vi "Autonomous Independent.vi"() -> ()   [LabVIEW 2014]
doc: "This VI is called when autonomous begins, and will automatically be terminated when autonomous ends. You can carry out timed or sensor driven robot movement independently without needing to return to the caller."
uses:
  <vilib>/Rock Robotics/WPI/SafetyOutput/WPI_SafetyOutputConfigMenu.ctl
  <vilib>/Rock Robotics/WPI/Joystick/WPI_JoystickGetSetRefNum.vi
  <vilib>/Rock Robotics/Network Tables/SD Read Number.vi
  <vilib>/Rock Robotics/WPI/RobotDrive/WPI_RobotDriveGetSetRefNum.vi
  <vilib>/Rock Robotics/WPI/RobotDrive/WPI_RobotDriveArcadeDrive_Standard(NoSaturation).vi
panel:
  out "Current Movement, for debugging":T1 {"Y Joystick Value" scale=1.0..-1.0; "X Joystick Value" scale=-1.0..1.0}
  in  "Array of robot movements":T2(array[cluster]) {"Y Joystick Value" scale=1.0..-1.0; "X Joystick Value" scale=-1.0..1.0}
  # "Be sure to right-click and choose Data Operations>>Make Current Value default if you want to save the array values with the VI"
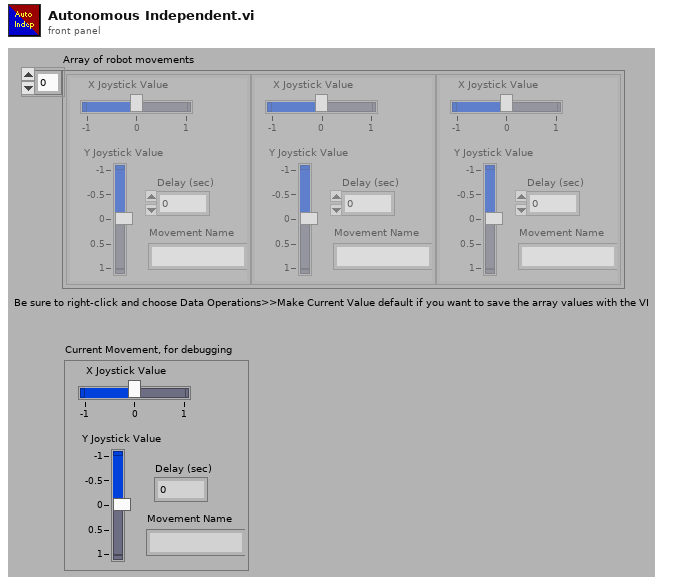
[diagram p1: front panel]
types:
  T1 = cluster{"X Joystick Value":dbl, "Y Joystick Value":dbl, "Delay (sec)":dbl, "Movement Name":string}
  T2 = cluster{"X Joystick Value":dbl, "Y Joystick Value":dbl, "Delay (sec)":dbl, "Movement Name":string}[]
  T3 = typedef "WPI_SafetyOutputConfigMenu.ctl" = enum16{"Enable", "Disable"}
  T4 = typedef "WPI_RobotDriveDevRef.ctl" = cluster{"DevStatus":errorcluster, "Motors[]":T5[], "Square Inputs":bool, "Max Output":dbl}
  T5 = typedef "WPI_MotorControlDeviceRef.ctl" = cluster{"DeviceStatus":errorcluster, "Type":T6, "PWM":cluster{"Controller":T7, "PWM Channel":T8, "DeadBand":T9}, "CAN":cluster{"Device Number":u8, "Control Mode":T10, "Semaphore":T11, "Max Vout":dbl, "TalonSRX Control Mode":T12}, "Invert":bool, "TransformRef":T13, "InvTransformRef":T13}
  T6 = typedef "WPI_MotorControlType.ctl" = enum16{"PWM", "CAN", "CANTalonSRX"}
  T7 = typedef "FPGA_TypedefDigitalModule.ctl" = enum16{"Controller 1"}
  T8 = typedef "FPGA_DIOPWMChannel.ctl" = enum8{"PWM 0", "PWM 1", "PWM 2", "PWM 3", "PWM 4", "PWM 5", "PWM 6", "PWM 7", "PWM 8", "PWM 9", "PWM MXP 0", "PWM MXP 1", "PWM MXP 2", "PWM MXP 3", "PWM MXP 4", "PWM MXP 5", "PWM MXP 6", "PWM MXP 7", "PWM MXP 8", "PWM MXP 9", "Invalid"}
  T9 = typedef "WPI_PWMDeadband.ctl" = cluster{"Name":string, "maxPositivePwm":i32, "minPositivePwm":i32, "centerPwm":i32, "maxNegativePwm":i32, "minNegativePwm":i32, "angularRange":u16}
  T10 = typedef "WPI_CANJaguar_ControlMode.ctl" = enum8{"Percent VBus", "Current", "Speed", "Position", "Voltage"}
  T11 = typedef "Semaphore RefNum" = refnum<k1>
  T12 = typedef "WPI_CANTalonSRX_APIControlMode.ctl" = enum8{"Percent VBus", "Speed", "Position", "Slave", "Unchanged / Invalid"}
  T13 = typedef "WPI_PWMTransform_ConPane.ctl" = refnum<vi>
  T14 = typedef "WPI_JoystickDevRef.ctl" = cluster{"Device":T15}
  T15 = typedef "WPI_JoystickDeviceEnum.ctl" = enum16{"USB 0", "USB 1", "USB 2", "USB 3", "USB 4", "USB 5"}
  T16 = typedef "WPI_GyroDevRef.ctl" = cluster{"DevStatus":errorcluster, "Analog Module":T17, "Analog Channel":T18, "Offset":dbl, "Gain (VoltsPerDegree/Second)":dbl}
  T17 = typedef "FPGA_TypedefAnalogModule.ctl" = enum16{"Controller 1"}
  T18 = typedef "FPGA_AIChannel.ctl" = enum8{"AI 0", "AI 1", "AI 2", "AI 3", "AI MXP 0", "AI MXP 1", "AI MXP 2", "AI MXP 3", "Invalid"}
  T19 = typedef "WPI_DigitalInputDevRef.ctl" = cluster{"DevStatus":errorcluster, "DIO Channel":T20, "Controller":T7}
  T20 = typedef "FPGA_DIOChannel.ctl" = enum8{"DIO 0", "DIO 1", "DIO 2", "DIO 3", "DIO 4", "DIO 5", "DIO 6", "DIO 7", "DIO 8", "DIO 9", "DIO MXP 0", "DIO MXP 1", "DIO MXP 2", "DIO MXP 3", "DIO MXP 4", "DIO MXP 5", "DIO MXP 6", "DIO MXP 7", "DIO MXP 8", "DIO MXP 9", "DIO MXP 10", "DIO MXP 11", "DIO MXP 12", "DIO MXP 13", "DIO MXP 14", "DIO MXP 15", "Invalid"}
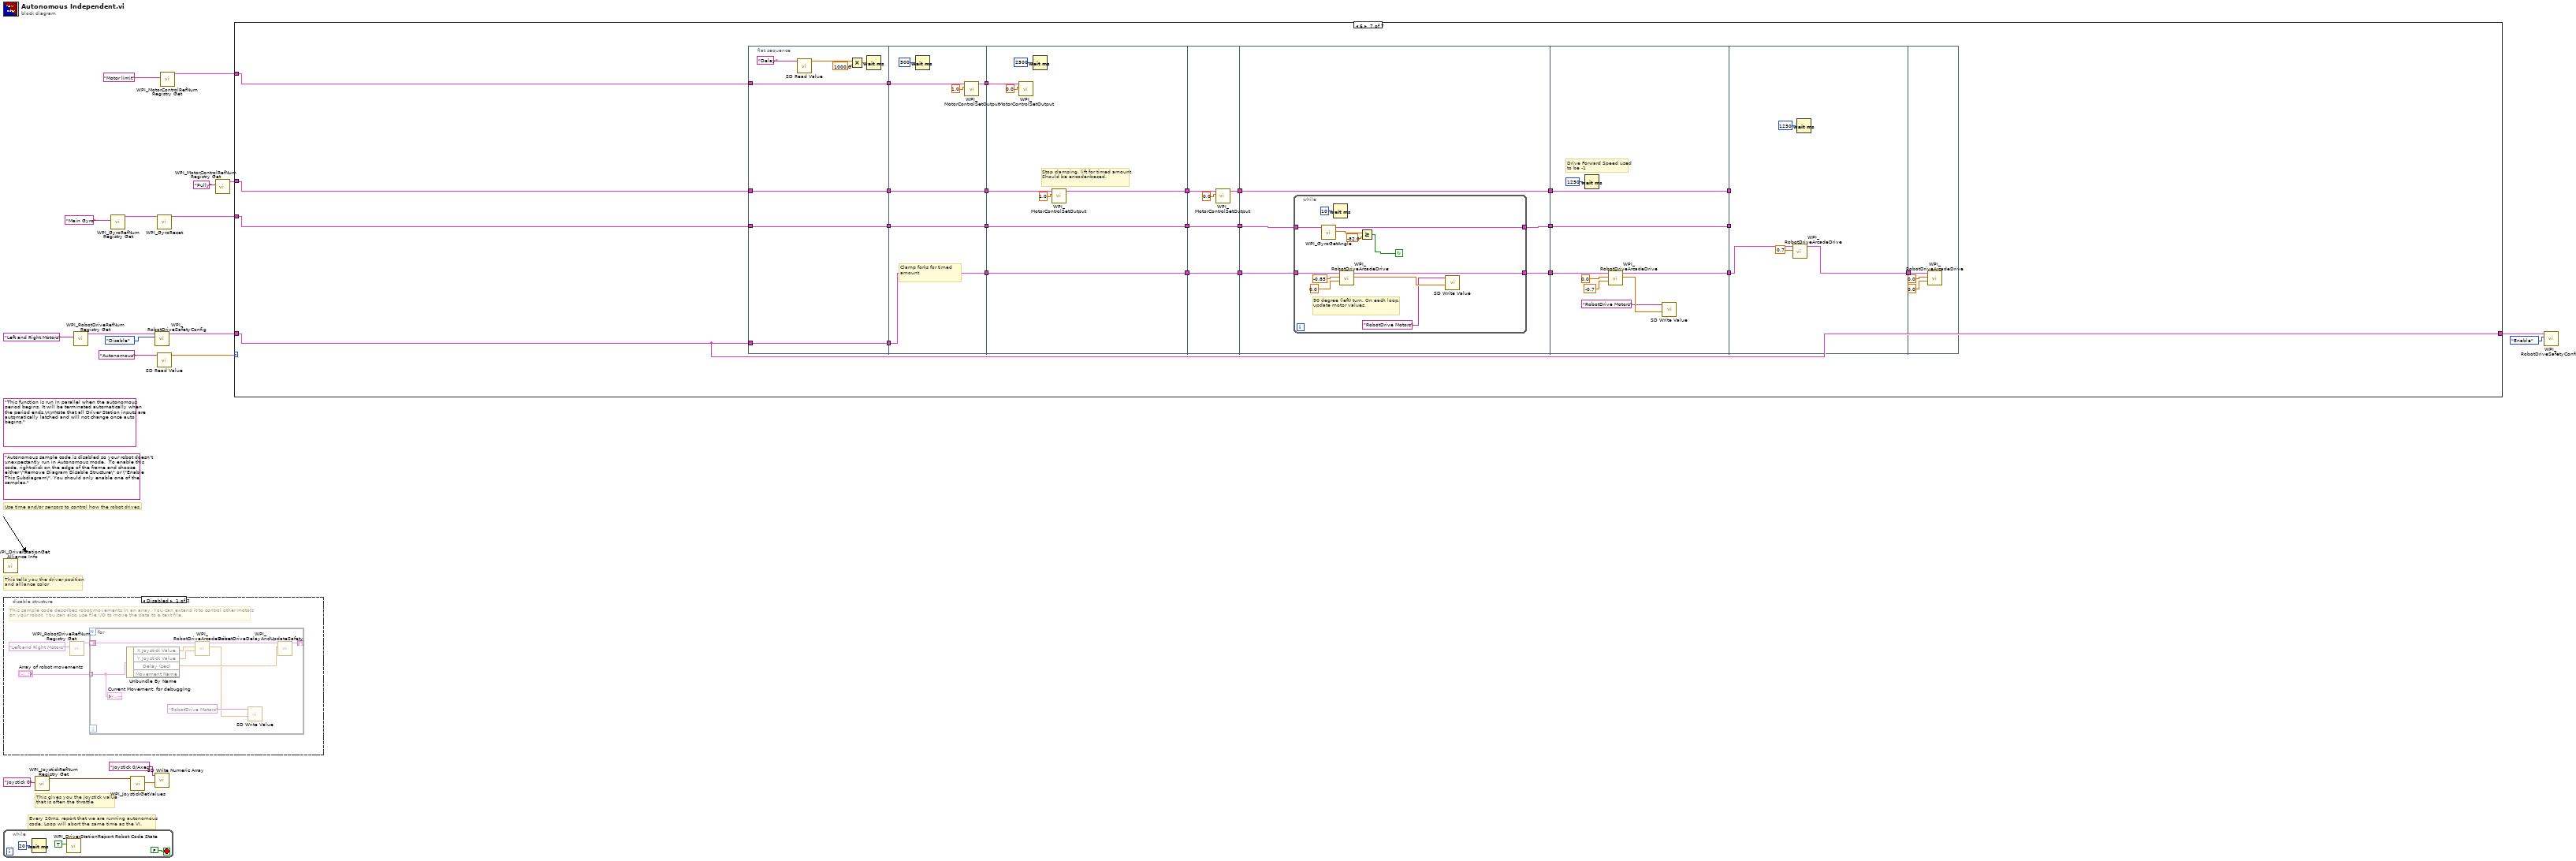
[diagram p0: block diagram]
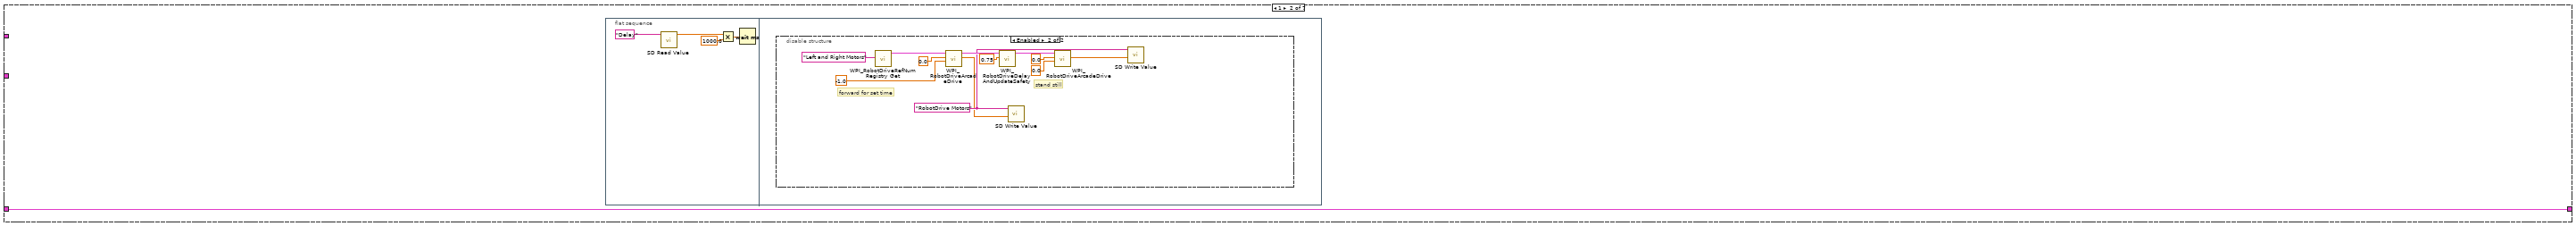
[diagram p3: hidden frame]
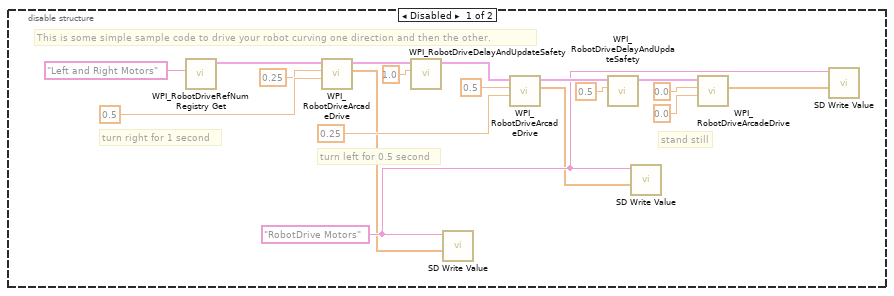
[diagram p4: hidden frame]
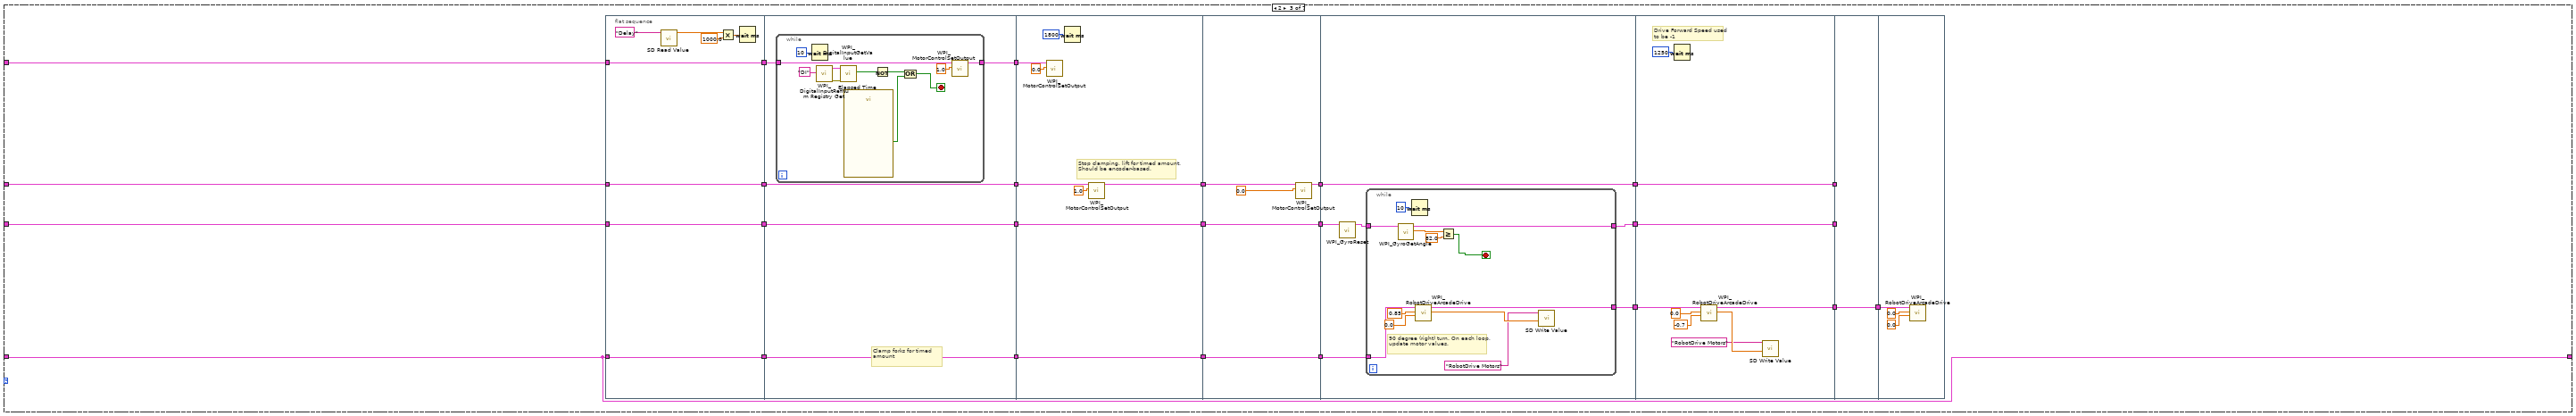
[diagram p5: hidden frame]
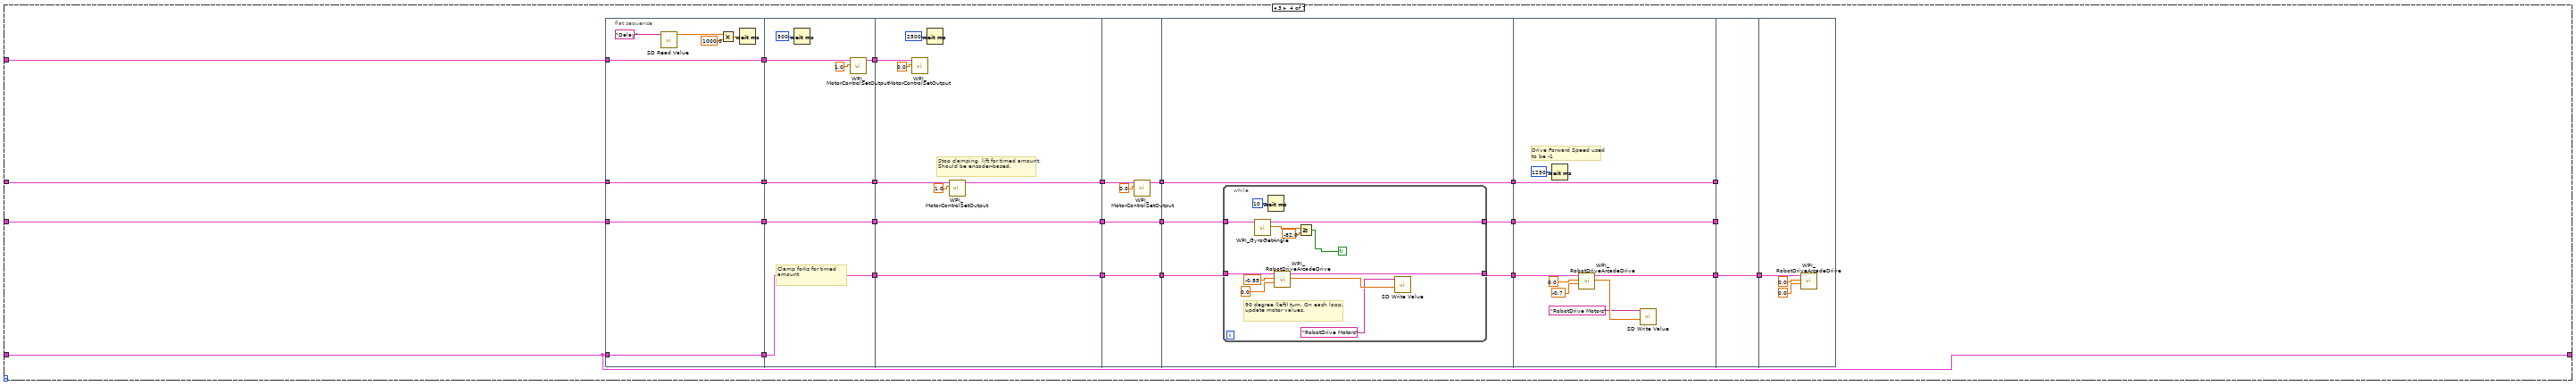
[diagram p6: hidden frame]
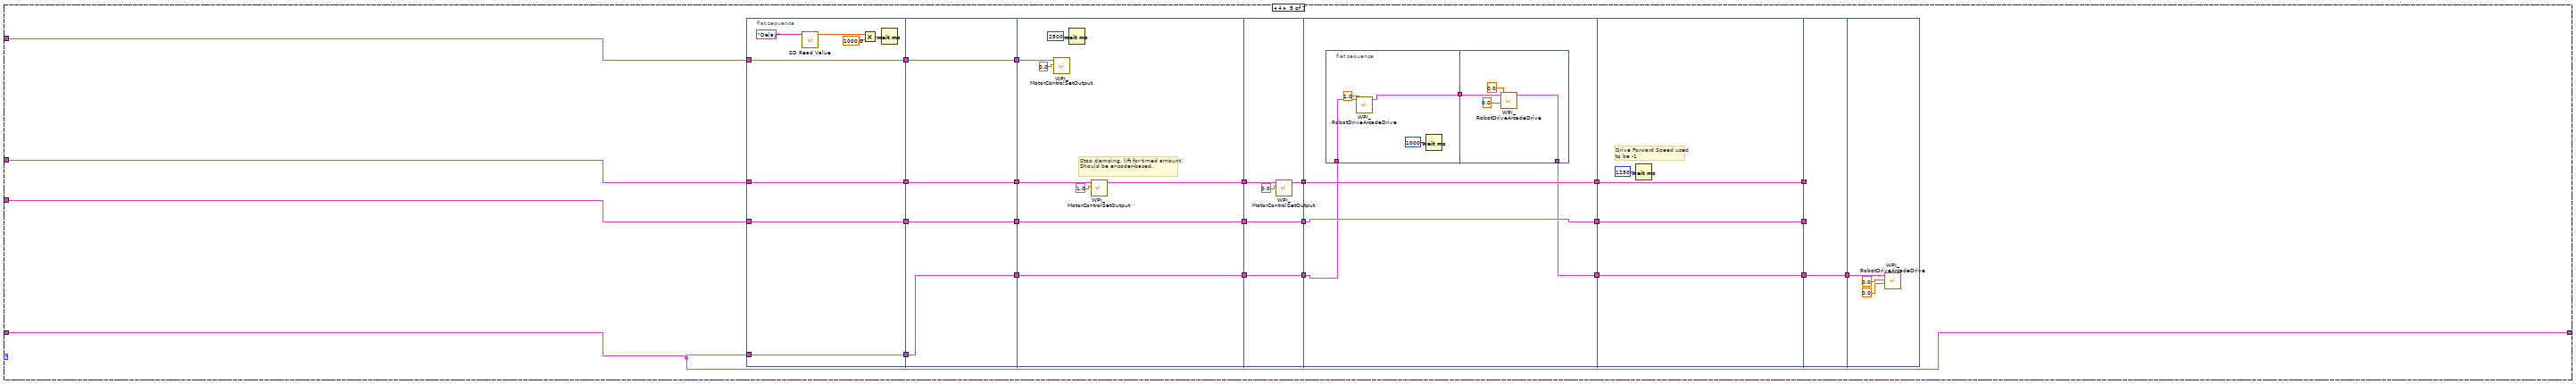
[diagram p7: hidden frame]
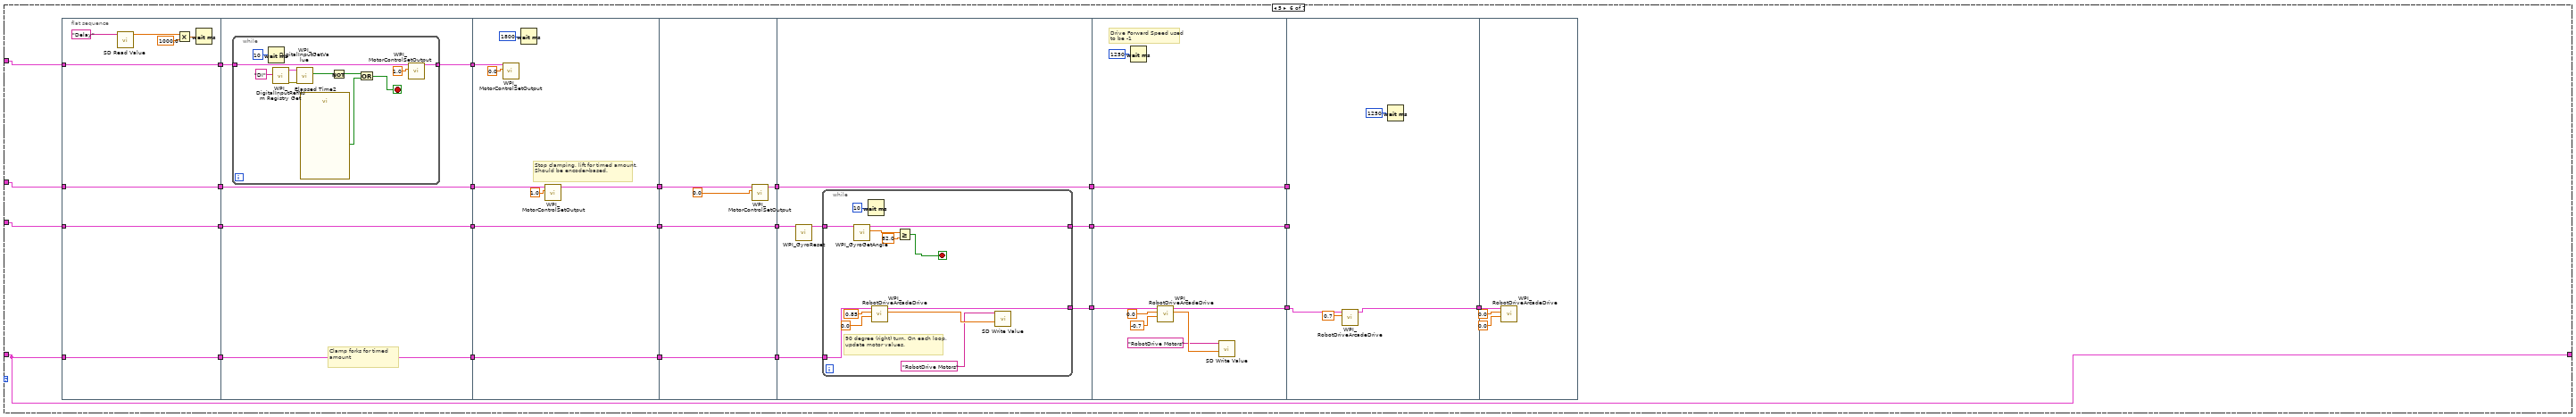
[diagram p8: hidden frame]
diagram:
  (unwired) "Autonomous sample code is disabled so your robot doesn't unexpectantly run in Autonomous mode.  To enable this code, right-click on the edge of the frame and choose either \"Remove Diagram Disable Structure\" or \"Enable This Subdiagram\". You should only enable one of the samples."
  (unwired) "This function is run in parallel when the autonomous period begins. It will be terminated automatically when the period ends.\n\nNote that all Driver Station inputs are automatically latched and will not change once auto begins."
  # "Every 20ms, report that we are running autonomous\ncode. Loop will abort the same time as the VI."
  # "This gives you the joystick value\nthat is often the throttle"
  # "Use time and/or sensors to control how the robot drives."
  # "This tells you the driver position\nand alliance color"
  n1 = call <vilib>:"WPI_DriverStationGet Alliance Info.vi"() -> ()  [unwired: 12 out]
  n2 = disable-structure shown="Disabled" {
    frame Disabled {
      # "This sample code describes robot movements in an array. You can extend it to control other motors\non your robot. You can also use file I/O to move the data to a text file."
      n3 = call <vilib>:"WPI_RobotDriveRefNum Registry Get.vi"("refnum name"="Left and Right Motors") -> ("RobotDriveDevRef"=w21:T4)  [unwired: 1 in, 9 out]
      n4 = for {
        shift-right: [w28] -> _
        shift-left: w21 -> [w29]
        tunnel: "Array of robot movements" -> [w24] mode=indexing
        n5 = Unbundle By Name(w24) -> ("X Joystick Value"=w27:dbl, "Y Joystick Value"=w26:dbl, "Delay (sec)"=w25:dbl)  [unwired: 1 out]
        n6 = call-poly <vilib>:"WPI_RobotDriveArcadeDrive.vi"("Y axis value"=w26, "X axis value"=w27, "RobotDriveDevRef"=w29) -> ("Motor Values"=w23:dbl[], "RobotDriveDevRef"=w30:T4)  [unwired: 1 in, 6 out]
        n7 = call-poly <vilib>:"SD Write Value.vi"("Numeric Array"=w23, "Name"="RobotDrive Motors") -> ()  [unwired: 8 in, 2 out]
        n8 = call <vilib>:"WPI_RobotDriveDelayAndUpdateSafety.vi"("Delay (s)"=w25, "RobotDriveDevRef"=w30) -> ("RobotDriveDevRef 2"=w28:T4)  [unwired: 8 in, 1 out]
        "Current Movement, for debugging" <- w24
      }
    }
    frame Enabled {
    }
  }
  n9 = while {
    stop <- FALSE stop-if-true
    n10 = Wait (ms)(milliseconds to wait=u32 20) -> ()  [unwired: 1 out]
    n11 = call <vilib>:"WPI_DriverStationReport Robot Code State.vi"("Autonomous"=TRUE) -> ()  [unwired: 10 in, 1 out]
  }
  n12 = call <vilib>:"WPI_JoystickRefNum Registry Get.vi"("refnum name"="Joystick 0") -> ("JoystickDevRef"=w18:T14)  [unwired: 1 in, 9 out]
  n13 = call <vilib>:"WPI_RobotDriveRefNum Registry Get.vi"("refnum name"="Left and Right Motors") -> ("RobotDriveDevRef"=w5:T4)  [unwired: 1 in, 9 out]
  n14 = call <vilib>:"WPI_GyroRefNum Registry Get.vi"("refnum name"="Main Gyro") -> ("GyroDevRef"=w12:T16)  [unwired: 9 in, 1 out]
  n15 = call <vilib>:"WPI_JoystickGetValues.vi"("JoystickDevRef"=w18) -> ("Axes"=w16:dbl[])  [unwired: 6 in, 4 out]
  n16 = call <vilib>:"SD Write Numeric Array.vi"("Numeric Array"=w16, "Name"="Joystick 0/Axes") -> ()  [unwired: 8 in, 2 out]
  n17 = call <vilib>:"WPI_RobotDriveSafetyConfig.vi"("mode"=WPI_SafetyOutputConfigMenu."Disable", "RobotDriveDevRef"=w5) -> ("RobotDriveDevRef"=w9:T4)  [unwired: 8 in, 1 out]
  n18 = call <vilib>:"WPI_GyroReset.vi"("GyroDevRef"=w12) -> ("GyroDevRef"=w11:T16)  [unwired: 9 in, 1 out]
  n19 = call-poly <vilib>:"SD Read Value.vi"("Name"="Autonomous") -> ("Numeric"=w14:dbl)  [unwired: 8 in, 2 out]
  n20 = call <vilib>:"WPI_MotorControlRefNum Registry Get.vi"("refnum name"="Motor limit") -> ("MotorControlDevRef"=w3:T5)  [unwired: 9 in, 1 out]
  n21 = call <vilib>:"WPI_MotorControlRefNum Registry Get.vi"("refnum name"="Pully") -> ("MotorControlDevRef"=w1:T5)  [unwired: 9 in, 1 out]
  n22 = case shown="6" w14 {
    tunnel: w11 -> [_ _ w77 w164 w249 w321 w416]
    tunnel: w9 -> [w35 w36 w74 w167 w250 w318 w417]
    tunnel: [w35 w36 w74 w167 w250 w318 w417] -> w8
    tunnel: w3 -> [_ _ w76 w165 w247 w319 w414]
    tunnel: w1 -> [_ _ w75 w166 w248 w320 w415]
    frame 0, Default {
    }
    frame 1 {
      n23 = flat-sequence {
        frame #0 {
          n24 = call-poly <vilib>:"SD Read Value.vi"("Name"="Delay") -> ("Numeric"=w40:dbl)  [unwired: 8 in, 2 out]
          n25 = Multiply(x=w40, y=1000.0) -> (x*y=w38:dbl)
          n26 = Wait (ms)(milliseconds to wait=w38) -> ()  [unwired: 1 out]
        }
        frame #1 {
          n27 = disable-structure shown="Enabled" {
            frame Disabled {
              w44 = "RobotDrive Motors" ("Name")
              # "This is some simple sample code to drive your robot curving one direction and then the other."
              # "stand still"
              # "turn left for 0.5 second"
              # "turn right for 1 second"
              n28 = call <vilib>:"WPI_RobotDriveRefNum Registry Get.vi"("refnum name"="Left and Right Motors") -> ("RobotDriveDevRef"=w45:T4)  [unwired: 1 in, 9 out]
              n29 = call-poly <vilib>:"WPI_RobotDriveArcadeDrive.vi"("Y axis value"=0.5 ("X axis value"), "X axis value"=0.25, "RobotDriveDevRef"=w45) -> ("Motor Values"=w43:dbl[], "RobotDriveDevRef"=w52:T4)  [unwired: 1 in, 6 out]
              n30 = call <vilib>:"WPI_RobotDriveDelayAndUpdateSafety.vi"("Delay (s)"=1.0, "RobotDriveDevRef"=w52) -> ("RobotDriveDevRef 2"=w51:T4)  [unwired: 8 in, 1 out]
              n31 = call-poly <vilib>:"SD Write Value.vi"("Numeric Array"=w43, "Name"=w44) -> ()  [unwired: 8 in, 2 out]
              n32 = call-poly <vilib>:"WPI_RobotDriveArcadeDrive.vi"("Y axis value"=0.25 ("X axis value"), "X axis value"=0.5, "RobotDriveDevRef"=w51) -> ("Motor Values"=w42:dbl[], "RobotDriveDevRef"=w50:T4)  [unwired: 1 in, 6 out]
              n33 = call <vilib>:"WPI_RobotDriveDelayAndUpdateSafety.vi"("Delay (s)"=0.5, "RobotDriveDevRef"=w50) -> ("RobotDriveDevRef 2"=w49:T4)  [unwired: 8 in, 1 out]
              n34 = call-poly <vilib>:"SD Write Value.vi"("Numeric Array"=w42, "Name"=w44) -> ()  [unwired: 8 in, 2 out]
              n35 = call-poly <vilib>:"WPI_RobotDriveArcadeDrive.vi"("Y axis value"=0.0 ("X axis value"), "X axis value"=0.0, "RobotDriveDevRef"=w49) -> ("Motor Values"=w41:dbl[])  [unwired: 1 in, 7 out]
              n36 = call-poly <vilib>:"SD Write Value.vi"("Numeric Array"=w41, "Name"=w44) -> ()  [unwired: 8 in, 2 out]
            }
            frame Enabled {
              w62 = "RobotDrive Motors" ("Name")
              # "stand still"
              # "forward for set time"
              n37 = call <vilib>:"WPI_RobotDriveRefNum Registry Get.vi"("refnum name"="Left and Right Motors") -> ("RobotDriveDevRef"=w63:T4)  [unwired: 1 in, 9 out]
              n38 = call-poly <vilib>:"WPI_RobotDriveArcadeDrive.vi"("Y axis value"=-1.0 ("X axis value"), "X axis value"=0.0, "RobotDriveDevRef"=w63) -> ("Motor Values"=w61:dbl[], "RobotDriveDevRef"=w66:T4)  [unwired: 1 in, 6 out]
              n39 = call <vilib>:"WPI_RobotDriveDelayAndUpdateSafety.vi"("Delay (s)"=0.75, "RobotDriveDevRef"=w66) -> ("RobotDriveDevRef 2"=w59:T4)  [unwired: 8 in, 1 out]
              n40 = call-poly <vilib>:"SD Write Value.vi"("Numeric Array"=w61, "Name"=w62) -> ()  [unwired: 8 in, 2 out]
              n41 = call-poly <vilib>:"WPI_RobotDriveArcadeDrive.vi"("Y axis value"=0.0 ("X axis value"), "X axis value"=0.0, "RobotDriveDevRef"=w59) -> ("Motor Values"=w60:dbl[])  [unwired: 1 in, 7 out]
              n42 = call-poly <vilib>:"SD Write Value.vi"("Numeric Array"=w60, "Name"=w62) -> ()  [unwired: 8 in, 2 out]
            }
          }
        }
      }
    }
    frame 2 {
      n43 = flat-sequence {
        tunnel: [w99] -> w95
        tunnel: [w96] -> w94
        tunnel: [w98] -> w93
        tunnel: [w97] -> w92
        tunnel: w77 -> [w99]
        tunnel: w76 -> [w98]
        tunnel: w75 -> [w97]
        tunnel: w74 -> [w96]
        tunnel: [w108] -> w91
        tunnel: [w104] -> w90
        tunnel: [w107] -> w89
        tunnel: [w106] -> w88
        tunnel: w95 -> [w108]
        tunnel: w94 -> [w107]
        tunnel: w93 -> [w105]
        tunnel: w92 -> [w106]
        tunnel: w91 -> [w125]
        tunnel: [w125] -> w87
        tunnel: w90 -> [w124]
        tunnel: [w122] -> w86
        tunnel: [w121] -> w85
        tunnel: w89 -> [w121]
        tunnel: w88 -> [w120]
        tunnel: w87 -> [w132]
        tunnel: [w132] -> w84
        tunnel: w86 -> [w131]
        tunnel: [w129] -> w83
        tunnel: w85 -> [w129]
        tunnel: [w128] -> w82
        tunnel: w84 -> [w134]
        tunnel: w83 -> [w138]
        tunnel: [w137] -> w81
        tunnel: [w136] -> w80
        tunnel: w82 -> [w136]
        tunnel: [w135] -> w71
        tunnel: [w154] -> w79
        tunnel: w81 -> [w153]
        tunnel: w80 -> [w152]
        tunnel: [w152] -> w78
        tunnel: [w151] -> w72
        tunnel: w71 -> [w151]
        tunnel: w78 -> [_]
        tunnel: w79 -> [w160]
        tunnel: [w160] -> w73
        tunnel: w72 -> [_]
        tunnel: w73 -> [w163]
        frame #0 {
          n44 = call-poly <vilib>:"SD Read Value.vi"("Name"="Delay") -> ("Numeric"=w103:dbl)  [unwired: 8 in, 2 out]
          n45 = Multiply(x=w103, y=1000.0) -> (x*y=w101:dbl)
          n46 = Wait (ms)(milliseconds to wait=w101) -> ()  [unwired: 1 out]
        }
        frame #1 {
          # "Clamp forks for timed amount"
          n47 = while {
            tunnel: w105 -> [w118]
            tunnel: [w117] -> w104
            stop <- w112 stop-if-true
            n48 = Wait (ms)(milliseconds to wait=u32 10) -> ()  [unwired: 1 out]
            n49 = call <vilib>:"WPI_DigitalInputRefNum Registry Get.vi"("refnum name"="DI") -> ("error out"=w116:errorcluster, "DigitalInputDevRef"=w115:T19)  [unwired: 9 in]
            n50 = call <vilib>:"WPI_DigitalInputGetValue.vi"("error in (no error)"=w116, "DigitalInputDevRef"=w115) -> ("Value"=w111:bool)  [unwired: 7 in, 2 out]
            n51 = call "Elapsed Time"() -> ("Time has Elapsed"=w113:bool)  [unwired: 12 in, 7 out]
            n52 = Not(x=w111) -> (.not. x?=w110:bool)
            n53 = Or(x=w110, y=w113) -> (x .or. y?=w112:bool)
            n54 = call <vilib>:"WPI_MotorControlSetOutput.vi"("Output"=1.0, "MotorControlDevRef"=w118) -> ("MotorControlDevRef"=w117:T5)  [unwired: 7 in, 2 out]
          }
        }
        frame #2 {
          # "Stop clamping, lift for timed amount. Should be encoder-based."
          n55 = call <vilib>:"WPI_MotorControlSetOutput.vi"("Output"=0.0, "MotorControlDevRef"=w124) -> ()  [unwired: 7 in, 3 out]
          n56 = Wait (ms)(milliseconds to wait=u32 1800) -> ()  [unwired: 1 out]
          n57 = call <vilib>:"WPI_MotorControlSetOutput.vi"("Output"=1.0, "MotorControlDevRef"=w120) -> ("MotorControlDevRef"=w122:T5)  [unwired: 7 in, 2 out]
        }
        frame #3 {
          n58 = call <vilib>:"WPI_MotorControlSetOutput.vi"("Output"=0.0, "MotorControlDevRef"=w131) -> ("MotorControlDevRef"=w128:T5)  [unwired: 7 in, 2 out]
        }
        frame #4 {
          n59 = call <vilib>:"WPI_GyroReset.vi"("GyroDevRef"=w134) -> ("GyroDevRef"=w133:T16)  [unwired: 9 in, 1 out]
          n60 = while {
            tunnel: w133 -> [w150]
            tunnel: w138 -> [w144]
            tunnel: [w143] -> w137
            tunnel: [w142] -> w135
            stop <- w139 stop-if-true
            # "90 degree (right) turn. On each loop, update motor values."
            n61 = call <vilib>:"WPI_GyroGetAngle.vi"("GyroDevRef"=w150) -> ("Angle"=w140:dbl, "GyroDevRef"=w142:T16)  [unwired: 7 in, 2 out]
            n62 = Wait (ms)(milliseconds to wait=u32 10) -> ()  [unwired: 1 out]
            n63 = call-poly <vilib>:"WPI_RobotDriveArcadeDrive.vi"("Y axis value"=0.0 ("X axis value"), "X axis value"=0.85, "RobotDriveDevRef"=w144) -> ("Motor Values"=w146:dbl[], "RobotDriveDevRef"=w143:T4)  [unwired: 1 in, 6 out]
            n64 = Greater Or Equal?(x=w140, y=82.0) -> (x >= y?=w139:bool)
            n65 = call-poly <vilib>:"SD Write Value.vi"("Numeric Array"=w146, "Name"="RobotDrive Motors") -> ()  [unwired: 8 in, 2 out]
          }
        }
        frame #5 {
          # "Drive Forward Speed used to be -1"
          n66 = Wait (ms)(milliseconds to wait=u32 1250) -> ()  [unwired: 1 out]
          n67 = call-poly <vilib>:"WPI_RobotDriveArcadeDrive.vi"("Y axis value"=-0.7, "X axis value"=0.0, "RobotDriveDevRef"=w153) -> ("Motor Values"=w157:dbl[], "RobotDriveDevRef"=w154:T4)  [unwired: 1 in, 6 out]
          n68 = call-poly <vilib>:"SD Write Value.vi"("Numeric Array"=w157, "Name"="RobotDrive Motors") -> ()  [unwired: 8 in, 2 out]
        }
        frame #6 {
        }
        frame #7 {
          n69 = call-poly <vilib>:"WPI_RobotDriveArcadeDrive.vi"("Y axis value"=0.0, "X axis value"=0.0, "RobotDriveDevRef"=w163) -> ()  [unwired: 1 in, 8 out]
        }
      }
    }
    frame 3 {
      n70 = flat-sequence {
        tunnel: [w192] -> w188
        tunnel: [w189] -> w187
        tunnel: [w191] -> w186
        tunnel: [w190] -> w185
        tunnel: w164 -> [w192]
        tunnel: w165 -> [w191]
        tunnel: w166 -> [w190]
        tunnel: w167 -> [w189]
        tunnel: [w201] -> w184
        tunnel: [w200] -> w183
        tunnel: [w199] -> w182
        tunnel: [w197] -> w181
        tunnel: w188 -> [w201]
        tunnel: w187 -> [w199]
        tunnel: w186 -> [w198]
        tunnel: w185 -> [w197]
        tunnel: w184 -> [w209]
        tunnel: [w209] -> w180
        tunnel: w183 -> [w208]
        tunnel: [w206] -> w179
        tunnel: [w205] -> w178
        tunnel: w182 -> [w205]
        tunnel: w181 -> [w204]
        tunnel: w180 -> [w216]
        tunnel: [w216] -> w177
        tunnel: w179 -> [w215]
        tunnel: [w213] -> w176
        tunnel: w178 -> [w213]
        tunnel: [w212] -> w175
        tunnel: w177 -> [w221]
        tunnel: w176 -> [w220]
        tunnel: [w219] -> w174
        tunnel: [w218] -> w173
        tunnel: w175 -> [w218]
        tunnel: [w217] -> w172
        tunnel: [w237] -> w170
        tunnel: w174 -> [w236]
        tunnel: w173 -> [w235]
        tunnel: [w235] -> w171
        tunnel: [w234] -> w169
        tunnel: w172 -> [w234]
        tunnel: w171 -> [_]
        tunnel: w170 -> [w243]
        tunnel: [w243] -> w168
        tunnel: w169 -> [_]
        tunnel: w168 -> [w246]
        frame #0 {
          n71 = call-poly <vilib>:"SD Read Value.vi"("Name"="Delay") -> ("Numeric"=w196:dbl)  [unwired: 8 in, 2 out]
          n72 = Multiply(x=w196, y=1000.0) -> (x*y=w194:dbl)
          n73 = Wait (ms)(milliseconds to wait=w194) -> ()  [unwired: 1 out]
        }
        frame #1 {
          # "Clamp forks for timed amount"
          n74 = Wait (ms)(milliseconds to wait=u32 500) -> ()  [unwired: 1 out]
          n75 = call <vilib>:"WPI_MotorControlSetOutput.vi"("Output"=1.0, "MotorControlDevRef"=w198) -> ("MotorControlDevRef"=w200:T5)  [unwired: 7 in, 2 out]
        }
        frame #2 {
          # "Stop clamping, lift for timed amount. Should be encoder-based."
          n76 = call <vilib>:"WPI_MotorControlSetOutput.vi"("Output"=0.0, "MotorControlDevRef"=w208) -> ()  [unwired: 7 in, 3 out]
          n77 = Wait (ms)(milliseconds to wait=u32 2500) -> ()  [unwired: 1 out]
          n78 = call <vilib>:"WPI_MotorControlSetOutput.vi"("Output"=1.0, "MotorControlDevRef"=w204) -> ("MotorControlDevRef"=w206:T5)  [unwired: 7 in, 2 out]
        }
        frame #3 {
          n79 = call <vilib>:"WPI_MotorControlSetOutput.vi"("Output"=0.0, "MotorControlDevRef"=w215) -> ("MotorControlDevRef"=w212:T5)  [unwired: 7 in, 2 out]
        }
        frame #4 {
          n80 = while {
            tunnel: w221 -> [w233]
            tunnel: w220 -> [w227]
            tunnel: [w226] -> w219
            tunnel: [w225] -> w217
            stop <- w222 continue-if-true
            # "90 degree (left) turn. On each loop, update motor values."
            n81 = call <vilib>:"WPI_GyroGetAngle.vi"("GyroDevRef"=w233) -> ("Angle"=w224:dbl, "GyroDevRef"=w225:T16)  [unwired: 7 in, 2 out]
            n82 = Wait (ms)(milliseconds to wait=u32 10) -> ()  [unwired: 1 out]
            n83 = call-poly <vilib>:"WPI_RobotDriveArcadeDrive.vi"("Y axis value"=0.0 ("X axis value"), "X axis value"=-0.85, "RobotDriveDevRef"=w227) -> ("Motor Values"=w229:dbl[], "RobotDriveDevRef"=w226:T4)  [unwired: 1 in, 6 out]
            n84 = Greater Or Equal?(x=w224, y=-82.0) -> (x >= y?=w222:bool)
            n85 = call-poly <vilib>:"SD Write Value.vi"("Numeric Array"=w229, "Name"="RobotDrive Motors") -> ()  [unwired: 8 in, 2 out]
          }
        }
        frame #5 {
          # "Drive Forward Speed used to be -1"
          n86 = Wait (ms)(milliseconds to wait=u32 1250) -> ()  [unwired: 1 out]
          n87 = call-poly <vilib>:"WPI_RobotDriveArcadeDrive.vi"("Y axis value"=-0.7, "X axis value"=0.0, "RobotDriveDevRef"=w236) -> ("Motor Values"=w240:dbl[], "RobotDriveDevRef"=w237:T4)  [unwired: 1 in, 6 out]
          n88 = call-poly <vilib>:"SD Write Value.vi"("Numeric Array"=w240, "Name"="RobotDrive Motors") -> ()  [unwired: 8 in, 2 out]
        }
        frame #6 {
        }
        frame #7 {
          n89 = call-poly <vilib>:"WPI_RobotDriveArcadeDrive.vi"("Y axis value"=0.0, "X axis value"=0.0, "RobotDriveDevRef"=w246) -> ()  [unwired: 1 in, 8 out]
        }
      }
    }
    frame 4 {
      n90 = flat-sequence {
        tunnel: [w275] -> w271
        tunnel: [w272] -> w270
        tunnel: [w274] -> w269
        tunnel: [w273] -> w268
        tunnel: w249 -> [w275]
        tunnel: w247 -> [w274]
        tunnel: w248 -> [w273]
        tunnel: w250 -> [w272]
        tunnel: [w283] -> w267
        tunnel: [w280] -> w266
        tunnel: [w282] -> w265
        tunnel: [w281] -> w264
        tunnel: w271 -> [w283]
        tunnel: w270 -> [w282]
        tunnel: w269 -> [w280]
        tunnel: w268 -> [w281]
        tunnel: w267 -> [w289]
        tunnel: [w289] -> w263
        tunnel: w266 -> [w288]
        tunnel: [w286] -> w262
        tunnel: [w285] -> w261
        tunnel: w265 -> [w285]
        tunnel: w264 -> [w284]
        tunnel: w263 -> [w296]
        tunnel: [w296] -> w260
        tunnel: w262 -> [w295]
        tunnel: [w293] -> w259
        tunnel: w261 -> [w293]
        tunnel: [w292] -> w258
        tunnel: w260 -> [w300]
        tunnel: w259 -> [w299]
        tunnel: [w297] -> w257
        tunnel: [w301] -> w256
        tunnel: w258 -> [w301]
        tunnel: [w300] -> w255
        tunnel: [w310] -> w253
        tunnel: w257 -> [w310]
        tunnel: w256 -> [w312]
        tunnel: [w312] -> w254
        tunnel: [w311] -> w252
        tunnel: w255 -> [w311]
        tunnel: w254 -> [_]
        tunnel: w253 -> [w314]
        tunnel: [w314] -> w251
        tunnel: w252 -> [_]
        tunnel: w251 -> [w317]
        frame #0 {
          n91 = call-poly <vilib>:"SD Read Value.vi"("Name"="Delay") -> ("Numeric"=w279:dbl)  [unwired: 8 in, 2 out]
          n92 = Multiply(x=w279, y=1000.0) -> (x*y=w277:dbl)
          n93 = Wait (ms)(milliseconds to wait=w277) -> ()  [unwired: 1 out]
        }
        frame #1 {
        }
        frame #2 {
          # "Stop clamping, lift for timed amount. Should be encoder-based."
          n94 = call <vilib>:"WPI_MotorControlSetOutput.vi"("Output"=0.0, "MotorControlDevRef"=w288) -> ()  [unwired: 7 in, 3 out]
          n95 = Wait (ms)(milliseconds to wait=u32 2500) -> ()  [unwired: 1 out]
          n96 = call <vilib>:"WPI_MotorControlSetOutput.vi"("Output"=1.0, "MotorControlDevRef"=w284) -> ("MotorControlDevRef"=w286:T5)  [unwired: 7 in, 2 out]
        }
        frame #3 {
          n97 = call <vilib>:"WPI_MotorControlSetOutput.vi"("Output"=0.0, "MotorControlDevRef"=w295) -> ("MotorControlDevRef"=w292:T5)  [unwired: 7 in, 2 out]
        }
        frame #4 {
          n98 = flat-sequence {
            tunnel: w299 -> [w305]
            tunnel: [w302] -> w298
            tunnel: w298 -> [w309]
            tunnel: [w306] -> w297
            frame #0 {
              n99 = call-poly <vilib>:"WPI_RobotDriveArcadeDrive.vi"("Y axis value"=1.0, "RobotDriveDevRef"=w305) -> ("RobotDriveDevRef"=w302:T4)  [unwired: 2 in, 7 out]
              n100 = Wait (ms)(milliseconds to wait=u32 1000) -> ()  [unwired: 1 out]
            }
            frame #1 {
              n101 = call-poly <vilib>:"WPI_RobotDriveArcadeDrive.vi"("Y axis value"=0.0, "X axis value"=0.0, "RobotDriveDevRef"=w309) -> ("RobotDriveDevRef"=w306:T4)  [unwired: 1 in, 7 out]
            }
          }
        }
        frame #5 {
          # "Drive Forward Speed used to be -1"
          n102 = Wait (ms)(milliseconds to wait=u32 1250) -> ()  [unwired: 1 out]
        }
        frame #6 {
        }
        frame #7 {
          n103 = call-poly <vilib>:"WPI_RobotDriveArcadeDrive.vi"("Y axis value"=0.0, "X axis value"=0.0, "RobotDriveDevRef"=w317) -> ()  [unwired: 1 in, 8 out]
        }
      }
    }
    frame 5 {
      n104 = flat-sequence {
        tunnel: [w346] -> w342
        tunnel: [w343] -> w341
        tunnel: [w345] -> w340
        tunnel: [w344] -> w339
        tunnel: w321 -> [w346]
        tunnel: w319 -> [w345]
        tunnel: w320 -> [w344]
        tunnel: w318 -> [w343]
        tunnel: [w355] -> w338
        tunnel: [w351] -> w337
        tunnel: [w354] -> w336
        tunnel: [w353] -> w335
        tunnel: w342 -> [w355]
        tunnel: w341 -> [w354]
        tunnel: w340 -> [w352]
        tunnel: w339 -> [w353]
        tunnel: w338 -> [w372]
        tunnel: [w372] -> w334
        tunnel: w337 -> [w371]
        tunnel: [w369] -> w333
        tunnel: [w368] -> w332
        tunnel: w336 -> [w368]
        tunnel: w335 -> [w367]
        tunnel: w334 -> [w379]
        tunnel: [w379] -> w331
        tunnel: w333 -> [w378]
        tunnel: [w376] -> w330
        tunnel: w332 -> [w376]
        tunnel: [w375] -> w329
        tunnel: w331 -> [w381]
        tunnel: w330 -> [w385]
        tunnel: [w384] -> w328
        tunnel: [w383] -> w327
        tunnel: w329 -> [w383]
        tunnel: [w382] -> w326
        tunnel: [w401] -> w324
        tunnel: w328 -> [w400]
        tunnel: w327 -> [w399]
        tunnel: [w399] -> w325
        tunnel: [w398] -> w323
        tunnel: w326 -> [w398]
        tunnel: w325 -> [_]
        tunnel: w324 -> [w410]
        tunnel: [w409] -> w322
        tunnel: w323 -> [_]
        tunnel: w322 -> [w413]
        frame #0 {
          n105 = call-poly <vilib>:"SD Read Value.vi"("Name"="Delay") -> ("Numeric"=w350:dbl)  [unwired: 8 in, 2 out]
          n106 = Multiply(x=w350, y=1000.0) -> (x*y=w348:dbl)
          n107 = Wait (ms)(milliseconds to wait=w348) -> ()  [unwired: 1 out]
        }
        frame #1 {
          # "Clamp forks for timed amount"
          n108 = while {
            tunnel: w352 -> [w365]
            tunnel: [w364] -> w351
            stop <- w359 stop-if-true
            n109 = Wait (ms)(milliseconds to wait=u32 10) -> ()  [unwired: 1 out]
            n110 = call <vilib>:"WPI_DigitalInputRefNum Registry Get.vi"("refnum name"="DI") -> ("error out"=w363:errorcluster, "DigitalInputDevRef"=w362:T19)  [unwired: 9 in]
            n111 = call <vilib>:"WPI_DigitalInputGetValue.vi"("error in (no error)"=w363, "DigitalInputDevRef"=w362) -> ("Value"=w358:bool)  [unwired: 7 in, 2 out]
            n112 = call "Elapsed Time2"() -> ("Time has Elapsed"=w360:bool)  [unwired: 12 in, 7 out]
            n113 = Not(x=w358) -> (.not. x?=w357:bool)
            n114 = Or(x=w357, y=w360) -> (x .or. y?=w359:bool)
            n115 = call <vilib>:"WPI_MotorControlSetOutput.vi"("Output"=1.0, "MotorControlDevRef"=w365) -> ("MotorControlDevRef"=w364:T5)  [unwired: 7 in, 2 out]
          }
        }
        frame #2 {
          # "Stop clamping, lift for timed amount. Should be encoder-based."
          n116 = call <vilib>:"WPI_MotorControlSetOutput.vi"("Output"=0.0, "MotorControlDevRef"=w371) -> ()  [unwired: 7 in, 3 out]
          n117 = Wait (ms)(milliseconds to wait=u32 1800) -> ()  [unwired: 1 out]
          n118 = call <vilib>:"WPI_MotorControlSetOutput.vi"("Output"=1.0, "MotorControlDevRef"=w367) -> ("MotorControlDevRef"=w369:T5)  [unwired: 7 in, 2 out]
        }
        frame #3 {
          n119 = call <vilib>:"WPI_MotorControlSetOutput.vi"("Output"=0.0, "MotorControlDevRef"=w378) -> ("MotorControlDevRef"=w375:T5)  [unwired: 7 in, 2 out]
        }
        frame #4 {
          n120 = call <vilib>:"WPI_GyroReset.vi"("GyroDevRef"=w381) -> ("GyroDevRef"=w380:T16)  [unwired: 9 in, 1 out]
          n121 = while {
            tunnel: w380 -> [w397]
            tunnel: w385 -> [w391]
            tunnel: [w390] -> w384
            tunnel: [w389] -> w382
            stop <- w386 stop-if-true
            # "90 degree (right) turn. On each loop, update motor values."
            n122 = call <vilib>:"WPI_GyroGetAngle.vi"("GyroDevRef"=w397) -> ("Angle"=w387:dbl, "GyroDevRef"=w389:T16)  [unwired: 7 in, 2 out]
            n123 = Wait (ms)(milliseconds to wait=u32 10) -> ()  [unwired: 1 out]
            n124 = call-poly <vilib>:"WPI_RobotDriveArcadeDrive.vi"("Y axis value"=0.0 ("X axis value"), "X axis value"=0.85, "RobotDriveDevRef"=w391) -> ("Motor Values"=w393:dbl[], "RobotDriveDevRef"=w390:T4)  [unwired: 1 in, 6 out]
            n125 = Greater Or Equal?(x=w387, y=82.0) -> (x >= y?=w386:bool)
            n126 = call-poly <vilib>:"SD Write Value.vi"("Numeric Array"=w393, "Name"="RobotDrive Motors") -> ()  [unwired: 8 in, 2 out]
          }
        }
        frame #5 {
          # "Drive Forward Speed used to be -1"
          n127 = Wait (ms)(milliseconds to wait=u32 1250) -> ()  [unwired: 1 out]
          n128 = call-poly <vilib>:"WPI_RobotDriveArcadeDrive.vi"("Y axis value"=-0.7, "X axis value"=0.0, "RobotDriveDevRef"=w400) -> ("Motor Values"=w404:dbl[], "RobotDriveDevRef"=w401:T4)  [unwired: 1 in, 6 out]
          n129 = call-poly <vilib>:"SD Write Value.vi"("Numeric Array"=w404, "Name"="RobotDrive Motors") -> ()  [unwired: 8 in, 2 out]
        }
        frame #6 {
          n130 = call-poly <vilib>:"WPI_RobotDriveArcadeDrive.vi"("X axis value"=0.7, "RobotDriveDevRef"=w410) -> ("RobotDriveDevRef"=w409:T4)  [unwired: 2 in, 7 out]
          n131 = Wait (ms)(milliseconds to wait=u32 1250) -> ()  [unwired: 1 out]
        }
        frame #7 {
          n132 = call-poly <vilib>:"WPI_RobotDriveArcadeDrive.vi"("Y axis value"=0.0, "X axis value"=0.0, "RobotDriveDevRef"=w413) -> ()  [unwired: 1 in, 8 out]
        }
      }
    }
    frame 6 {
      n133 = flat-sequence {
        tunnel: [w442] -> w438
        tunnel: [w439] -> w437
        tunnel: [w441] -> w436
        tunnel: [w440] -> w435
        tunnel: w416 -> [w442]
        tunnel: w414 -> [w441]
        tunnel: w415 -> [w440]
        tunnel: w417 -> [w439]
        tunnel: [w451] -> w434
        tunnel: [w450] -> w433
        tunnel: [w449] -> w432
        tunnel: [w447] -> w431
        tunnel: w438 -> [w451]
        tunnel: w437 -> [w449]
        tunnel: w436 -> [w448]
        tunnel: w435 -> [w447]
        tunnel: w434 -> [w459]
        tunnel: [w459] -> w430
        tunnel: w433 -> [w458]
        tunnel: [w456] -> w429
        tunnel: [w455] -> w428
        tunnel: w432 -> [w455]
        tunnel: w431 -> [w454]
        tunnel: w430 -> [w466]
        tunnel: [w466] -> w427
        tunnel: w429 -> [w465]
        tunnel: [w463] -> w426
        tunnel: w428 -> [w463]
        tunnel: [w462] -> w425
        tunnel: w427 -> [w471]
        tunnel: w426 -> [w470]
        tunnel: [w469] -> w424
        tunnel: [w468] -> w423
        tunnel: w425 -> [w468]
        tunnel: [w467] -> w422
        tunnel: [w487] -> w420
        tunnel: w424 -> [w486]
        tunnel: w423 -> [w485]
        tunnel: [w485] -> w421
        tunnel: [w484] -> w419
        tunnel: w422 -> [w484]
        tunnel: w421 -> [_]
        tunnel: w420 -> [w496]
        tunnel: [w495] -> w418
        tunnel: w419 -> [_]
        tunnel: w418 -> [w499]
        frame #0 {
          n134 = call-poly <vilib>:"SD Read Value.vi"("Name"="Delay") -> ("Numeric"=w446:dbl)  [unwired: 8 in, 2 out]
          n135 = Multiply(x=w446, y=1000.0) -> (x*y=w444:dbl)
          n136 = Wait (ms)(milliseconds to wait=w444) -> ()  [unwired: 1 out]
        }
        frame #1 {
          # "Clamp forks for timed amount"
          n137 = Wait (ms)(milliseconds to wait=u32 500) -> ()  [unwired: 1 out]
          n138 = call <vilib>:"WPI_MotorControlSetOutput.vi"("Output"=1.0, "MotorControlDevRef"=w448) -> ("MotorControlDevRef"=w450:T5)  [unwired: 7 in, 2 out]
        }
        frame #2 {
          # "Stop clamping, lift for timed amount. Should be encoder-based."
          n139 = call <vilib>:"WPI_MotorControlSetOutput.vi"("Output"=0.0, "MotorControlDevRef"=w458) -> ()  [unwired: 7 in, 3 out]
          n140 = Wait (ms)(milliseconds to wait=u32 2500) -> ()  [unwired: 1 out]
          n141 = call <vilib>:"WPI_MotorControlSetOutput.vi"("Output"=1.0, "MotorControlDevRef"=w454) -> ("MotorControlDevRef"=w456:T5)  [unwired: 7 in, 2 out]
        }
        frame #3 {
          n142 = call <vilib>:"WPI_MotorControlSetOutput.vi"("Output"=0.0, "MotorControlDevRef"=w465) -> ("MotorControlDevRef"=w462:T5)  [unwired: 7 in, 2 out]
        }
        frame #4 {
          n143 = while {
            tunnel: w471 -> [w483]
            tunnel: w470 -> [w477]
            tunnel: [w476] -> w469
            tunnel: [w475] -> w467
            stop <- w472 continue-if-true
            # "90 degree (left) turn. On each loop, update motor values."
            n144 = call <vilib>:"WPI_GyroGetAngle.vi"("GyroDevRef"=w483) -> ("Angle"=w474:dbl, "GyroDevRef"=w475:T16)  [unwired: 7 in, 2 out]
            n145 = Wait (ms)(milliseconds to wait=u32 10) -> ()  [unwired: 1 out]
            n146 = call-poly <vilib>:"WPI_RobotDriveArcadeDrive.vi"("Y axis value"=0.0 ("X axis value"), "X axis value"=-0.85, "RobotDriveDevRef"=w477) -> ("Motor Values"=w479:dbl[], "RobotDriveDevRef"=w476:T4)  [unwired: 1 in, 6 out]
            n147 = Greater Or Equal?(x=w474, y=-82.0) -> (x >= y?=w472:bool)
            n148 = call-poly <vilib>:"SD Write Value.vi"("Numeric Array"=w479, "Name"="RobotDrive Motors") -> ()  [unwired: 8 in, 2 out]
          }
        }
        frame #5 {
          # "Drive Forward Speed used to be -1"
          n149 = Wait (ms)(milliseconds to wait=u32 1250) -> ()  [unwired: 1 out]
          n150 = call-poly <vilib>:"WPI_RobotDriveArcadeDrive.vi"("Y axis value"=-0.7, "X axis value"=0.0, "RobotDriveDevRef"=w486) -> ("Motor Values"=w490:dbl[], "RobotDriveDevRef"=w487:T4)  [unwired: 1 in, 6 out]
          n151 = call-poly <vilib>:"SD Write Value.vi"("Numeric Array"=w490, "Name"="RobotDrive Motors") -> ()  [unwired: 8 in, 2 out]
        }
        frame #6 {
          n152 = call-poly <vilib>:"WPI_RobotDriveArcadeDrive.vi"("X axis value"=0.7, "RobotDriveDevRef"=w496) -> ("RobotDriveDevRef"=w495:T4)  [unwired: 2 in, 7 out]
          n153 = Wait (ms)(milliseconds to wait=u32 1250) -> ()  [unwired: 1 out]
        }
        frame #7 {
          n154 = call-poly <vilib>:"WPI_RobotDriveArcadeDrive.vi"("Y axis value"=0.0, "X axis value"=0.0, "RobotDriveDevRef"=w499) -> ()  [unwired: 1 in, 8 out]
        }
      }
    }
  }
  n155 = call <vilib>:"WPI_RobotDriveSafetyConfig.vi"("mode"=WPI_SafetyOutputConfigMenu."Enable", "RobotDriveDevRef"=w8) -> ()  [unwired: 8 in, 2 out]
